vi "Shoot Select Mode.vi"() -> (3 "Auton Shooter Command":T1)   [LabVIEW 2019]
uses:
  .Team Code/Robot Global Data.vi
  Shooter Mode Type Def.ctl
  Shooter Command Type Def.ctl
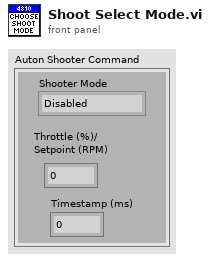
[diagram p1: front panel]
types:
  T1 = typedef "Shooter Command Type Def.ctl" = cluster{"Shooter Mode":T2, "Throttle (%)/ \nSetpoint (RPM)":dbl, "Timestamp (ms)":dbl}
  T2 = typedef "Shooter Mode Type Def.ctl" = enum16{"Disabled", "Raw Throttle", "Velocity Control"}
  T3 = typedef "WPI_DriverStationRobotMode2.ctl" = enum16{"Autonomous Disabled", "Autonomous Enabled", "Teleop Disabled", "Teleop Enabled", "Disconnected", "Finish", "Test Disabled", "Test Enabled", "Emergency Stopped"}
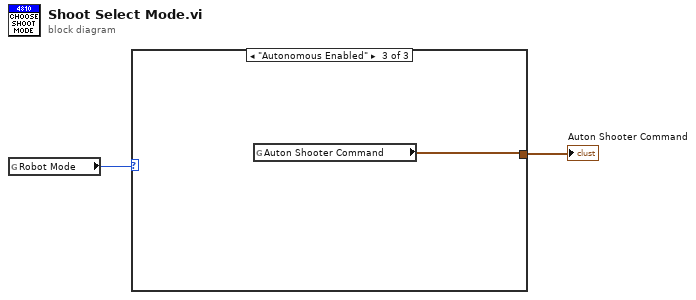
[diagram p0: block diagram]
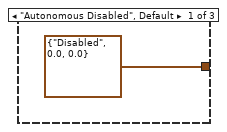
[diagram p2: hidden frame]
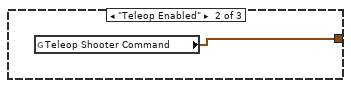
[diagram p3: hidden frame]
diagram:
  n1 = global read "Robot Global Data.vi" "Robot Mode"() -> (w2:T3)
  n2 = case shown="\"Autonomous Enabled\"" w2 {
    tunnel: [T1 {"Shooter Mode"=enum."Disabled", "Throttle (%)/ \nSetpoint (RPM)"=0.0, "Timestamp (ms)"=0.0} ("Teleop Shooter Command") w4 w5] -> w1
    frame "Autonomous Disabled", Default {
    }
    frame "Teleop Enabled" {
      n3 = global read "Robot Global Data.vi" "Teleop Shooter Command"() -> (w4:T1)
    }
    frame "Autonomous Enabled" {
      n4 = global read "Robot Global Data.vi" "Auton Shooter Command"() -> (w5:T1)
    }
  }
  "Auton Shooter Command" <- w1
